vi "Initialize-object.vi"(7 "Heartbeat interval":dbl, 8 "error in (no error)":errorcluster, 9 "Client channel":refnum<queue>, 10 "Server channel":refnum<queue>) -> (0 "error out":errorcluster, 3 "Reference out":T1)   [LabVIEW 2013, in "Module-communication.lvlib" / "Client.lvclass"]
uses:
  Client.lvclass
  Object-reference.ctl
  Messages/Message.lvclass
  Client.lvclass/Client.ctl
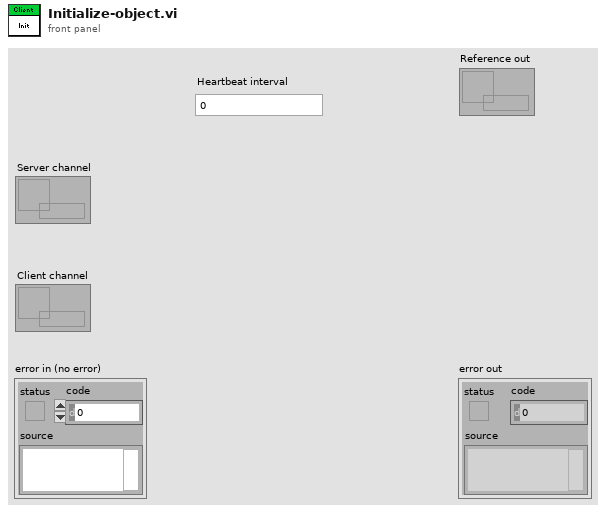
[diagram p1: front panel]
types:
  T1 = typedef "Module-communication.lvlib/Client.lvclass/Object-reference.ctl" = refnum<data-value>
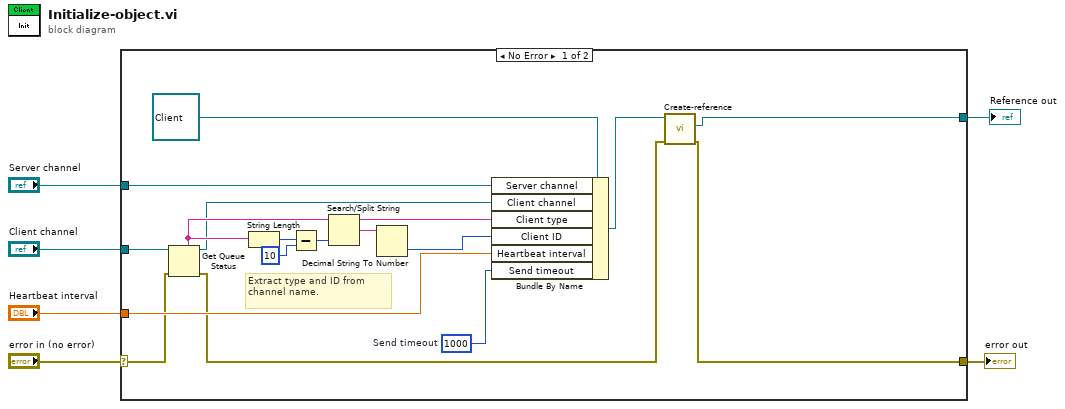
[diagram p0: block diagram]
diagram:
  n1 = case shown="No Error" "error in (no error)" {
    selector: "error in (no error)" -> [w11 w25]
    tunnel: [w24 w25] -> w5
    tunnel: [w23 _] -> w4
    tunnel: "Heartbeat interval" -> [w22 _]
    tunnel: "Client channel" -> [w21 _]
    tunnel: "Server channel" -> [w13 _]
    frame No Error {
      w7 = 1000  # Send timeout
      # "Extract type and ID from\nchannel name."
      n2 = Get Queue Status(queue=w21, error in (no error)=w11) -> (queue out=w12:refnum<queue>, queue name=w17:string, error out=w10:errorcluster)  [unwired: 1 in, 5 out]
      n3 = String Length(string=w17) -> (length=w20:i32)
      n4 = Subtract(x=w20, y=10) -> (x-y=w18:i32)
      n5 = Search/Split String(string=w17, offset (0)=w18) -> (substring before match=w14:string, match + rest of string=w16:string)  [unwired: 1 in, 1 out]
      n6 = Decimal String To Number(string=w16) -> (number=w15:i32)  [unwired: 2 in, 1 out]
      n7 = Bundle By Name(cluster=refnum<class "Client.lvclass"> refnum ("Panes.lvclass"), "Server channel"=w13, "Client channel"=w12, "Client type"=w14, "Client ID"=w15, "Heartbeat interval"=w22, "Send timeout"=w7) -> (w8:refnum<class "Client.lvclass">)
      n8 = call "Create-reference.vi"("error in (no error)"=w10, "Object in"=w8) -> ("error out"=w24:errorcluster, "Object reference"=w23:T1)  [unwired: 7 in, 1 out]
    }
    frame Error {
    }
  }
  "error out" <- w5
  "Reference out" <- w4
